vi "Networked Temperature Monitor RT Host.vi"() -> ()   [LabVIEW 2010]
uses:
  <vilib>/userDefined/High Color/nirio_resource_hc.ctl
  <vilib>/rvi/interface/nirviOpenFPGA/nirviOpenFPGA.xnode
  FPGA Bitfiles/TemperatureMonit_FPGATarget_TemperatureMonit_0C4E9FD6.lvbitx
  Temperature Monitor FPGA.vi
  <vilib>/rvi/ClientSDK/nirviWhatTheDeviceIsDoing.ctl
  <vilib>/rvi/interface/nirviReadWriteControl/nirviReadWriteControl.xnode
  <vilib>/rvi/interface/common/niFpgaNodeNameForErrorReporting.ctl
  <vilib>/rvi/errors/niLvFpgaWhatHappensToTopLevelVI.ctl
  <vilib>/rvi/interface/nirviCloseFPGA/nirviCloseFPGA.xnode
  <vilib>/FPGAPlugInAG/cRIO-9074/niLvFpga_Open_cRIO-9074.vi
  NI 9211 Support Files.llb/NI 9211 Convert to Temperature (Calibrated).vi
  <vilib>/Utility/error.llb/Error Cluster From Error Code.vi
  <vilib>/rvi/errors/niLvFpgaAdjustHostInterfaceError.vi
  <vilib>/FPGAPlugInAG/cRIO-9074/niLvFpga_Close_cRIO-9074.vi
  NiFpgaLv.dll
panel:
  in  "stop":bool
  out "Linearized\nTemperature (C)":sgl(graph) caption="Linearized Temperature (C)"
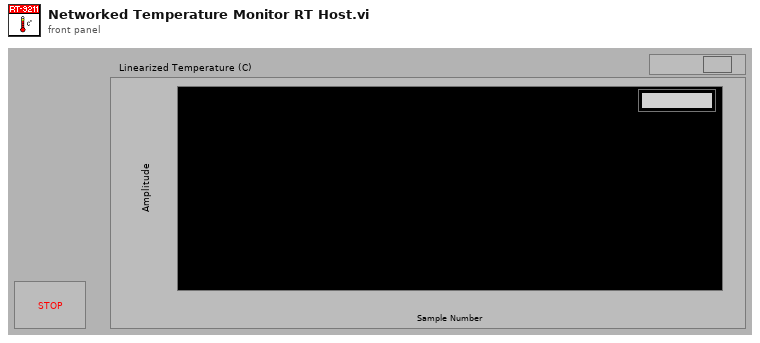
[diagram p1: front panel]
types:
  T1 = typedef "niFpgaNodeNameForErrorReporting.ctl" = enum16{"Open FPGA VI Reference", "Read/Write Control", "Invoke Method: Abort", "Invoke Method: Acknowledge IRQ", "Invoke Method: Download", "Invoke Method: FIFO.Configure", "Invoke Method: FIFO.Read", "Invoke Method: FIFO.Start", "Invoke Method: FIFO.Stop", "Invoke Method: FIFO.Write", "Invoke Method: Reset", "Invoke Method: Run", "Invoke Method: Wait on IRQ", "Close FPGA VI Reference"}
  T2 = typedef "niLvFpgaWhatHappensToTopLevelVI.ctl" = enum16{"top level VI scripted behind XNode", "top level VI inlined behind XNode"}
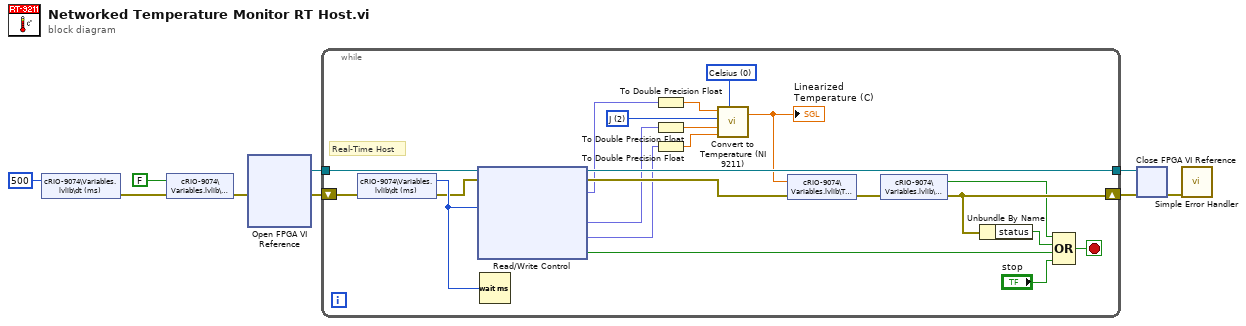
[diagram p0: block diagram]
diagram:
  n1 = shared-variable "cRIO-9074\\Variables.lvlib\\dt (ms)"(u32 500 ("dt (ms)")) -> (error out=w3:errorcluster)  [unwired: 1 out]
  n2 = shared-variable "cRIO-9074\\Variables.lvlib\\Stop"(FALSE ("Stop"), error in=w3) -> (error out=w4:errorcluster)
  n3 = xnode "Open FPGA VI Reference"("error in"=w4) -> ("FPGA VI Reference Out"=w9:refnum<k20>, "error out"=w8:errorcluster)  [unwired: 1 in]
  n4 = while {
    shift-right: [w21] -> w6
    shift-left: w8 -> [w24]
    tunnel: w9 -> [w31]
    tunnel: [w30] -> w7
    stop <- w27 stop-if-true
    w25 = u16 2 items=["B", "E", "J", "K", "R", "S", "T", "N", "IC (C)", "IC (F)", "Therm."] ("ThermocoupleType")
    w26 = u16 0 items=["Celsius", "Fahrenheit", "Kelvin", "Rankine"] ("Temperature Units (C)")
    # "Real-Time Host"
    n5 = shared-variable "cRIO-9074\\Variables.lvlib\\dt (ms)"(error in=w24) -> (w18:u32, error out=w17:errorcluster)
    n6 = xnode "Read/Write Control"("FPGA VI Reference In"=w31, "error in"=w17, "Sample Period (ms)"=w18) -> ("FPGA VI Reference Out"=w30:refnum<k20>, "error out"=w22:errorcluster, "Temperature"=w16:fxp<+/-,24,-2>, "CJC"=w14:fxp<+/-,24,-2>, "Autozero"=w13:fxp<+/-,24,-2>, "status"=w10:bool)
    n7 = Wait (ms)(milliseconds to wait=w18) -> ()  [unwired: 1 out]
    n8 = To Double Precision Float(number=w16) -> (double precision float=w15:dbl)
    n9 = To Double Precision Float(number=w14) -> (double precision float=w12:dbl)
    n10 = To Double Precision Float(number=w13) -> (double precision float=w11:dbl)
    n11 = call-poly "Convert to Temperature (NI 9211).vi"("Temperature Units (C)"=w26, "Autozero Channel"=w11, "CJC Channel"=w12, "ThermocoupleType"=w25, "Thermocouple Channel"=w15) -> ("Linearized Temperature"=w19:sgl)  [unwired: 2 out]
    "Linearized\nTemperature (C)" <- w19
    n12 = shared-variable "cRIO-9074\\Variables.lvlib\\T (C)"(w19, error in=w22) -> (error out=w23:errorcluster)
    n13 = shared-variable "cRIO-9074\\Variables.lvlib\\Stop"(error in=w23) -> (w20:bool, error out=w21:errorcluster)
    n14 = Unbundle By Name(w21) -> ("status"=w29:bool)
    n15 = Compound Arithmetic op=OR(w20, w29, w10, "stop") -> (w27:bool)
  }
  n16 = xnode "Close FPGA VI Reference"("FPGA VI Reference In"=w7, "error in"=w6) -> ("error out"=w5:errorcluster)
  n17 = call <vilib>:"Simple Error Handler.vi"("error in (no error)"=w5) -> ()  [unwired: 1 in, 8 out]
